vi "adam.vi"() -> ()   [LabVIEW 2013]
panel:
  out "Current position":dbl
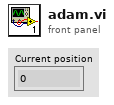
[diagram p1: front panel]
types:
  T1 = cluster{"VISA resource name":refnum<visa-resource-name>, "Device name":string, "Controller address":i32, "error":errorcluster}
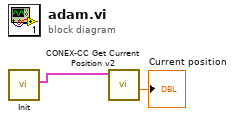
[diagram p0: block diagram]
diagram:
  n1 = call "Init.vi"() -> ("Device Connection Cluster"=w2:T1)  [unwired: 4 in, 3 out]
  n2 = call <userlib>:"CONEX-CC Get Current Position v2.vi"("Connection Cluster in"=w2) -> ("Current position"=→"Current position":dbl)  [unwired: 8 in, 2 out]
